vi "rate_of_rise_calc.vi"(3 "Temperature [C]":dbl, 5 "Pressure Rate [Pa/s]":dbl) -> (1 "Rate of Rise [sccm]":dbl)   [LabVIEW 2016]
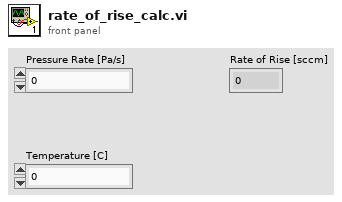
[diagram p1: front panel]
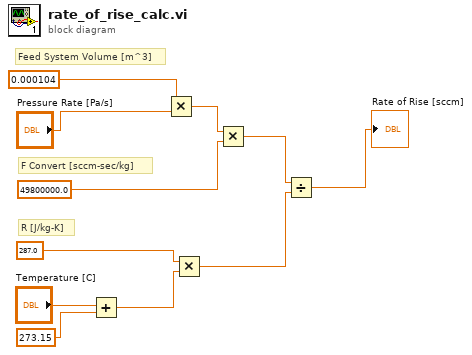
[diagram p0: block diagram]
diagram:
  # "Feed System Volume [m^3]"
  # "F Convert [sccm-sec/kg]"
  # "R [J/kg-K]"
  n1 = Add(x="Temperature [C]", y=273.15) -> (x+y=w3:dbl)
  n2 = Multiply(x=0.000104, y="Pressure Rate [Pa/s]") -> (x*y=w10:dbl)
  n3 = Multiply(x=287.0, y=w3) -> (x*y=w7:dbl)
  n4 = Multiply(x=w10, y=49800000.0) -> (x*y=w8:dbl)
  n5 = Divide(x=w8, y=w7) -> (x/y=→"Rate of Rise [sccm]":dbl)
